vi "Dequeue Message w timeout.vi"(8 "entrée d'erreur (pas d'erreur)":errorcluster, 10 "timeout en ms (-1)":i32=-1, 11 "Message Queue":refnum<queue>) -> (0 "sortie d'erreur":errorcluster, 1 "Message Data":variant, 2 "Message":string, 3 "Message Queue":refnum<queue>)   [LabVIEW 2024]
uses:
  Message Cluster.ctl
  Message Queue.lvlib
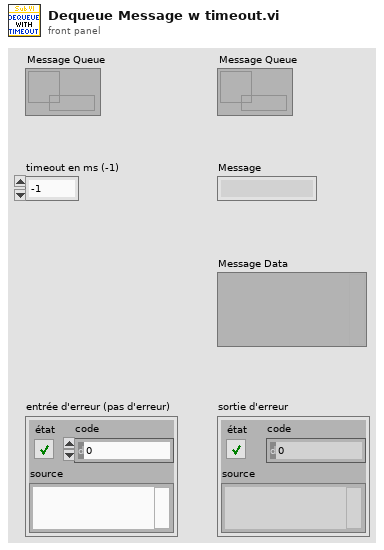
[diagram p1: front panel]
types:
  T1 = typedef "Message Queue.lvlib/Message Cluster.ctl" = cluster{"Message":string, "Message Data":variant}
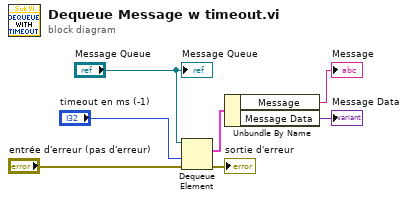
[diagram p0: block diagram]
diagram:
  n1 = Dequeue Element(queue="Message Queue", timeout in ms (-1)="timeout en ms (-1)", error in (no error)="entrée d'erreur (pas d'erreur)") -> (element=w4:T1, error out=→"sortie d'erreur":errorcluster)  [unwired: 2 out]
  n2 = Unbundle By Name(w4) -> ("Message"=→"Message":string, "Message Data"=→"Message Data":variant)
  "Message Queue" <- "Message Queue"
